vi "lua_remove.vi"(8 "error in (no error)":errorcluster, 10 "index":i32, 11 "lua_state_p":u64) -> (0 "error out":errorcluster, 3 "lua_state_p out":u64)   [LabVIEW 2020, in "lua.dll.lvlib"]
uses:
  lua.dll.lvlib
  lua_settop.vi
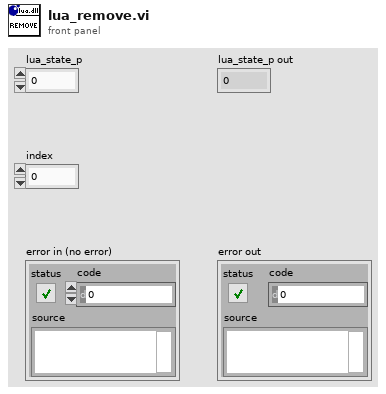
[diagram p1: front panel]
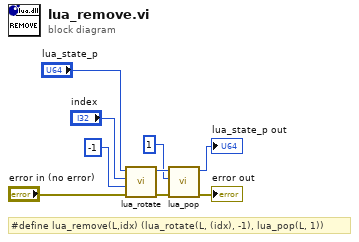
[diagram p0: block diagram]
diagram:
  # "#define lua_remove(L,idx)\t(lua_rotate(L, (idx), -1), lua_pop(L, 1))"
  n1 = call "lua_rotate.vi"("error in (no error)"="error in (no error)", "n"=-1, "index"="index", "lua_state_p"="lua_state_p") -> ("error out"=w9:errorcluster, "lua_state_p out"=w5:u64)  [unwired: 6 in]
  n2 = call "lua_pop.vi"("error in (no error)"=w9, "n"=1, "lua_state_p"=w5) -> ("error out"=→"error out":errorcluster, "lua_state_p out"=→"lua_state_p out":u64)  [unwired: 7 in]
